vi "Simple AAP.vi"() -> ()   [LabVIEW 2010]
doc: "This VI acquires, analyzes, and presents data. It is a solution VI to an exercise in the LabVIEW Core I course. Refer to the course manual for instructions."
uses:
  Instance           3 18Saved   Simple AAP .vi
  Instance           2 18Saved   Simple AAP .vi
panel:
  out "Average Value":dbl
  out "Waveform Graph":dynamicdata(graph)
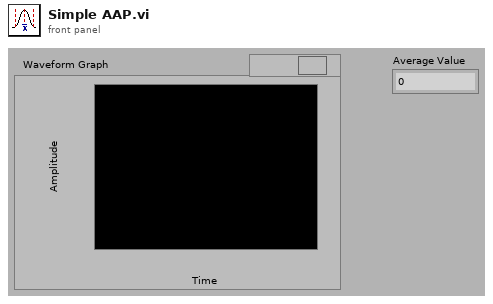
[diagram p1: front panel]
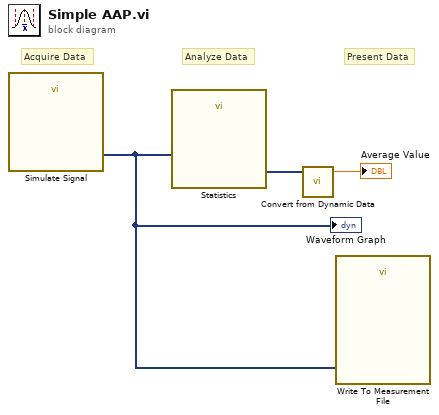
[diagram p0: block diagram]
diagram:
  # "Present Data"
  # "Analyze Data"
  # "Acquire Data"
  n1 = call "Simulate Signal"() -> ("Sine"=w3:dynamicdata)  [unwired: 14 in, 1 out]
  "Waveform Graph" <- w3
  n2 = call "Statistics"("Signals"=w3) -> ("Arithmetic Mean"=w2:dynamicdata)  [unwired: 25 in, 1 out]
  n3 = call "Convert from Dynamic Data"("Dynamic Data Type"=w2) -> ("Scalar"=→"Average Value":dbl)  [unwired: 3 in]
  n4 = call "Write To Measurement File"("Signals"=w3) -> ()  [unwired: 8 in, 3 out]
